vi "rqp_Set EHL Timeout.vi"(4 "Show in Debugger?":bool=TRUE, 6 "Message Priority":T1=enum."Normal", 7 "Caller in":refnum<class "Worker.lvclass">, 8 "error in":errorcluster, 9 "Data in":T2={"Timeout (ms)"=-1}, 11 "Message Pump in":refnum<class "_Message Pump.lvclass">) -> (0 "error out":errorcluster, 3 "dup Message Pump out":refnum<class "_Message Pump.lvclass">, 5 "dup Caller out":refnum<class "Worker.lvclass">)   [LabVIEW 2017, in "_Message Pump.lvclass"]
doc: "This VI sends a <b>Public API Request</b> message to an MHL case of the Worker that owns this VI.\n---\nSets the wait period (in ms) of the EHL's event timer"
uses:
  _Message Pump.lvclass
  C:/SC/Source Code/VIPM/LabVIEW 20xx/vi.lib/addons/_Workers/Library/Classes/Worker/Worker.lvclass
  <vilib>/addons/_Workers/Library/Classes/Worker/Worker.lvclass
  rqp_Set EHL Timeout.ctl
  <vilib>/addons/_Workers/Library/Classes/Message/Priority.ctl
  <vilib>/addons/_Workers/Library/Case Label.ctl
  <vilib>/addons/_Workers/Library/Classes/Message Queue/Message Queue.lvclass
  <vilib>/addons/_Workers/Library/Workers.lvlib
  <vilib>/addons/_Workers/Library/Classes/Message/Message.lvclass
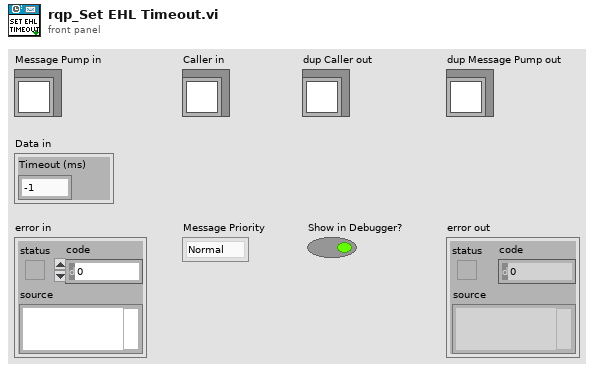
[diagram p1: front panel]
types:
  T1 = typedef "Workers.lvlib/Message.lvclass/Priority.ctl" = enum16{"Low", "Normal", "High"}
  T2 = typedef "_Message Pump.lvclass/rqp_Set EHL Timeout.ctl" = cluster{"Timeout (ms)":i32}
  T3 = typedef "Workers.lvlib/Case Label.ctl" = string
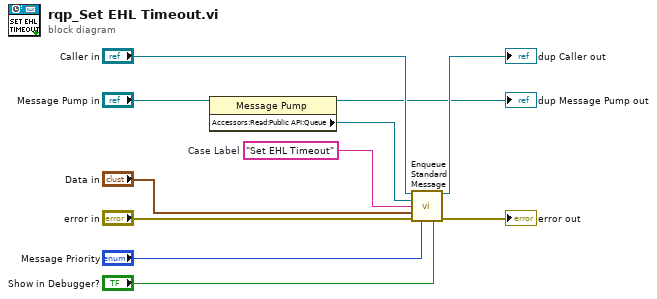
[diagram p0: block diagram]
diagram:
  w1 = T3 "Set EHL Timeout"  # Case Label
  n1 = property class="Message Pump"(reference="Message Pump in") -> (reference out=→"dup Message Pump out":refnum<class "_Message Pump.lvclass">, "Accessors:Read:Public API:Queue"=w2:refnum<class "Message Queue.lvclass">)  [unwired: 1 in, 1 out]
  n2 = call-dynamic "Enqueue Standard Message.vi"("Worker"="Caller in", "Message Queue"=w2, "Case Label"=w1, "Data"="Data in", "error in (no error)"="error in", "Priority (Normal)"="Message Priority", "Send Message to Debugger? (T)"="Show in Debugger?") -> ("dup Worker out"=→"dup Caller out":refnum<class "Worker.lvclass">, "error out"=→"error out":errorcluster)  [unwired: 7 in]
